vi "SetAMaxVMax.vi"(0 "handle in":i32, 1 "UnitAddress(0)":u16, 2 "MotNr(0)":u8, 5 "error in":errorcluster, 7 "VMaxAMax":T1={"VMax(511)"=511, "AMax(128)"=128}) -> (14 "handle out":i32, 19 "error out":errorcluster)   [LabVIEW 2014, in "Sixpack - Driver.lvlib"]
doc: "ACHTUNG: AMax und VMax werden permanent überprüft! Änderungen werden sofort behandelt!\n\nAMax gibt die Steigung der linearen Beschleunigungsrampe an. Ausgehend von VStart (Startgeschwindigkeit, siehe SetVMinVStart) wird VAkt (die aktuelle Geschwindigkeit, Abfrage über GetVelocityAndActivity) alle 2 ms um den festen Wert 1/64 * AMax inkrementiert. Wenn der nächste Erhöhungsschritt den Wert von VMax überschreiten würde, wird VAkt auf VMax gesetzt.\nVMax gibt den Wert für die Maximalgeschwindigkeit an. Nach welcher Formel sich die Geschwindigkeit berechnet, wird im Manual Kapitel 3.3.1 beschrieben.\n\nCMD $14\nMotorNr (0...5)\nAMax (1..32767): Maximale Beschleunigung des Motors.\n Funktionsweise: while (VAkt >= VMax) do VAkt = VAkt + ( AMax/64 );\n VAkt = VMax;\nVMax (1..511): Maximaler Wert für VAkt"
uses:
  Sixpack - Driver.lvlib
  VmaxAmax.ctl
  DLL/PackDLL.dll
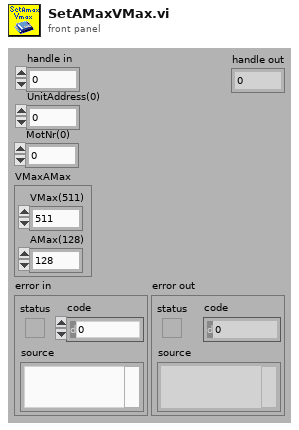
[diagram p1: front panel]
types:
  T1 = typedef "Sixpack - Driver.lvlib/VmaxAmax.ctl" = cluster{"VMax(511)":u16, "AMax(128)":u16}
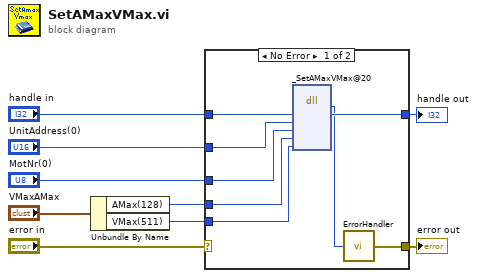
[diagram p0: block diagram]
diagram:
  n1 = Unbundle By Name("VMaxAMax") -> ("AMax(128)"=w2:u16, "VMax(511)"=w1:u16)
  n2 = case shown="No Error" "error in" {
    selector: "error in" -> [_ w18]
    tunnel: "handle in" -> [w17 w19]
    tunnel: [w16 w19] -> w8
    tunnel: "UnitAddress(0)" -> [w15 _]
    tunnel: "MotNr(0)" -> [w14 _]
    tunnel: w2 -> [w13 _]
    tunnel: w1 -> [w12 _]
    tunnel: [w10 w18] -> w4
    frame No Error {
      n3 = dll-call lib="D:/CS-Source/LV2014/GPL/instr.lib/SixPack/PackDLL/DLL/PackDLL.dll" fn="_SetAMaxVMax@20" label="SetAMaxVMax"("HANDLE"=w17, "UnitAddress"=w15, "MotNr"=w14, "AMax"=w13, "VMax"=w12) -> ("BOOLEAN"=w11:i8, "HANDLE"=w16:i32)  [unwired: 7 in, 2 out]
      n4 = call "ErrorHandler.vi"("BOOLEAN"=w11) -> ("error out"=w10:errorcluster)
    }
    frame Error {
    }
  }
  "handle out" <- w8
  "error out" <- w4
